vi "Z900_navX_Close.vi"(8 "error in (no error)":errorcluster, 11 "navX Device":T1={"Interface"={"Protocol"=enum."SERIAL", "Update Rate (4Hz-100Hz)"=4, "navX Open TypeDef"=variant}, "Notify Packet"=refnum, "Loop VI Refnum"=refnum, "Ready to Close Occurrence Refnum"=refnum} {"Interface"."Update Rate (4Hz-100Hz)" min=4 max=60 step=1}) -> (0 "error out":errorcluster)   [LabVIEW 2015, in "Apple Pi Gyro Library.lvlib" / "navX Library v2.lvlib"]
doc: "This navX VI closes the background processing loop and shutsdown any open interfaces used for the navX.\nTHIS VI SHOULD BE CALLED WHEN DONE.\nPLACE IT IN FINISH.VI"
uses:
  navX Library v2.lvlib
  TypeDefs/Z900_navX_DeviceTypeDef.ctl
  TypeDefs/Z900_navX_ProtocolTypeDef.ctl
  TypeDefs/Z900_navX_NotifyPacketTypeDef.ctl
  TypeDefs/Z900_navX_ActionTypeDef.ctl
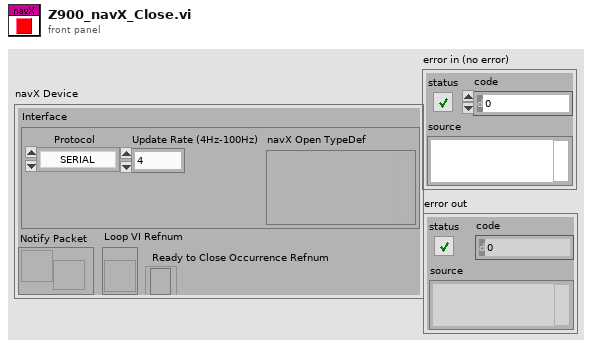
[diagram p1: front panel]
types:
  T1 = typedef "Apple Pi Gyro Library.lvlib/navX Library v2.lvlib/Z900_navX_DeviceTypeDef.ctl" = cluster{"Interface":cluster{"Protocol":T2, "Update Rate (4Hz-100Hz)":u8, "navX Open TypeDef":variant}, "Notify Packet":refnum<notifier>, "Loop VI Refnum":refnum<vi>, "Ready to Close Occurrence Refnum":refnum<k4>}
  T2 = typedef "Apple Pi Gyro Library.lvlib/navX Library v2.lvlib/Z900_navX_ProtocolTypeDef.ctl" = enum16{"SERIAL", "I2C", "SPI"}
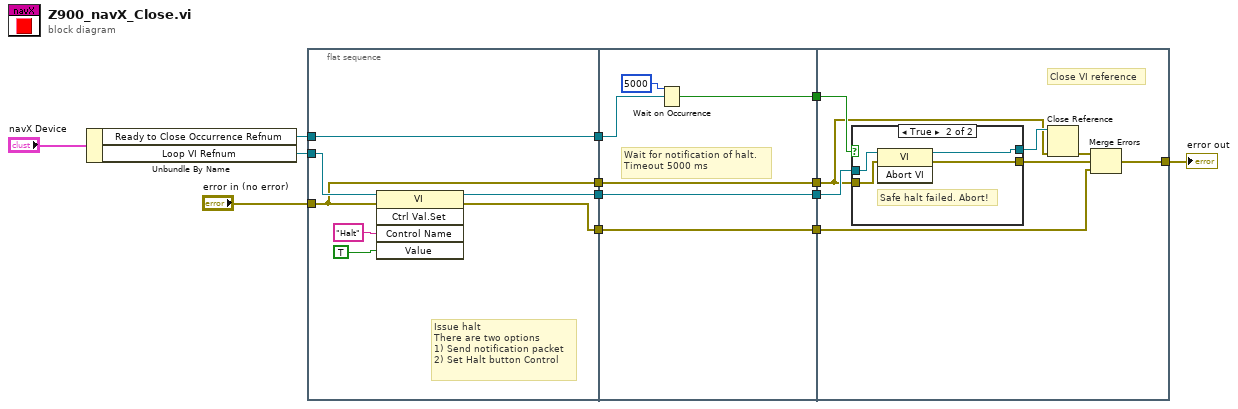
[diagram p0: block diagram]
diagram:
  n1 = Unbundle By Name("navX Device") -> ("Ready to Close Occurrence Refnum"=w1:refnum<k4>, "Loop VI Refnum"=w12:refnum<vi>)
  n2 = flat-sequence {
    tunnel: w12 -> [w20]
    tunnel: "error in (no error)" -> [w16]
    tunnel: [w18] -> w11
    tunnel: [w17] -> w7
    tunnel: w1 -> [w17]
    tunnel: [w16] -> w5
    tunnel: [w15] -> w3
    tunnel: w11 -> [w26]
    tunnel: [w26] -> w10
    tunnel: [w24] -> w8
    tunnel: w7 -> [w23]
    tunnel: [w22] -> w6
    tunnel: w5 -> [w22]
    tunnel: [w21] -> w4
    tunnel: w3 -> [w21]
    tunnel: w10 -> [w34]
    tunnel: [w30] -> w2
    tunnel: w8 -> [w29]
    tunnel: w6 -> [w28]
    tunnel: w4 -> [w27]
    frame #0 {
      # "Issue halt\nThere are two options\n1) Send notification packet\n2) Set Halt button Control"
      n3 = invoke class="VI" method="Ctrl Val.Set"(reference=w20, error in=w16, "Control Name"="Halt", "Value"=TRUE) -> (reference out=w18:refnum<vi>, error out=w15:errorcluster)  [unwired: 1 in, 3 out]
    }
    frame #1 {
      # "Wait for notification of halt.\nTimeout 5000 ms"
      n4 = Wait on Occurrence(2:w23, 3:5000 ("ms timeout (-1)")) -> (0:w24:bool)  [unwired: 1 in]
    }
    frame #2 {
      # "Close VI reference"
      n5 = case shown="True" w29 {
        tunnel: w34 -> [w35 w39]
        tunnel: [w35 w38] -> w33
        tunnel: [_ w37] -> w31
        tunnel: w28 -> [_ w36]
        frame False {
          # "Safe abort success"
        }
        frame True {
          # "Safe halt failed. Abort!"
          n6 = invoke class="VI" method="Abort VI"(reference=w39, error in=w36) -> (reference out=w38:refnum<vi>, error out=w37:errorcluster)  [unwired: 1 in, 1 out]
        }
      }
      n7 = Close Reference(reference=w33, error in (no error)=w28) -> (error out=w32:errorcluster)
      n8 = Merge Errors(w32, w31, w27) -> (w30:errorcluster)
    }
  }
  "error out" <- w2
